vi "strerror_r.vi"(8 "error in (no error)":errorcluster, 11 "errno":i32) -> (0 "error out":errorcluster, 3 "error string":string)   [LabVIEW 2013, in "Linux Errno.lvlib"]
doc: "Wrapper VI for glibc function strerror_r()."
uses:
  Linux Errno.lvlib
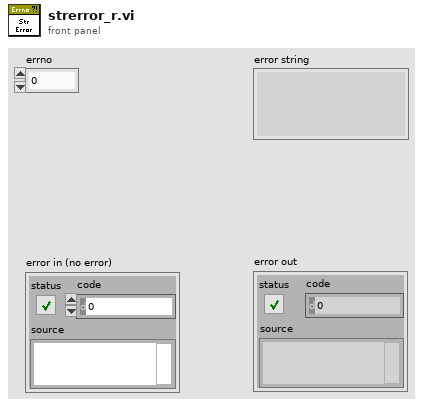
[diagram p1: front panel]
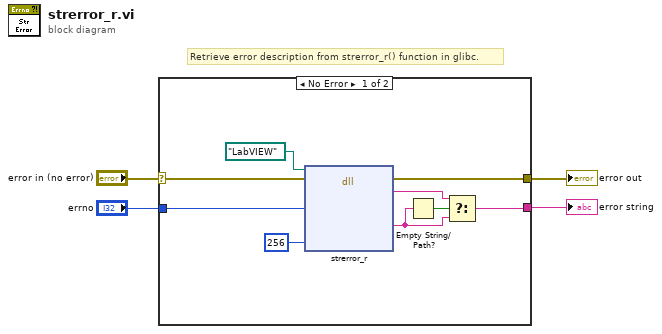
[diagram p0: block diagram]
diagram:
  # "Retrieve error description from strerror_r() function in glibc."
  n1 = case shown="No Error" "error in (no error)" {
    selector: "error in (no error)" -> [w6 w14]
    tunnel: [w13 w14] -> w3
    tunnel: [w12 _] -> w2
    tunnel: "errno" -> [w11 _]
    frame No Error {
      n2 = dll-call lib="?" fn="strerror_r"(path in=path "LabVIEW", error in=w6, "errnum"=w11, "string_len"=256) -> (error out=w13:errorcluster, "return"=w7:string, "string"=w8:string)  [unwired: 4 in, 1 out]
      n3 = Empty String/Path?(string/path=w8) -> (empty?=w9:bool)
      n4 = Select(t=w7, s=w9, f=w8) -> (s? t:f=w12:string)
    }
    frame Error {
    }
  }
  "error out" <- w3
  "error string" <- w2
